vi "Deaktivate HovaCAL MFC Komp fix.vi"(8 "error in (no error)":errorcluster caption="Fehler (Eingang, kein Fehler)", 11 "AutoLin MFC":i32) -> (0 "error out":errorcluster caption="Fehler (Ausgang)", 3 "AutoLin MFC out":i32)   [LabVIEW 2020, in "Linearisierung v2.lvlib" / "Gasteiler.lvlib" / "HovaCAL_Interface.lvlib" / "Helper.lvlib"]
uses:
  Helper.lvlib
  Kommunikation/Kommunikation.lvlib
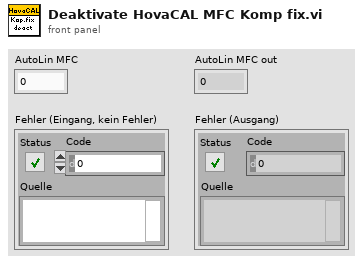
[diagram p1: front panel]
types:
  T1 = cluster{"MFC Komponenten Array":refnum<vi>[], "MFC fix + Array":refnum<vi>[]}
  T2 = enum8{"Enabled", "Disabled", "Disabled and Grayed Out"}
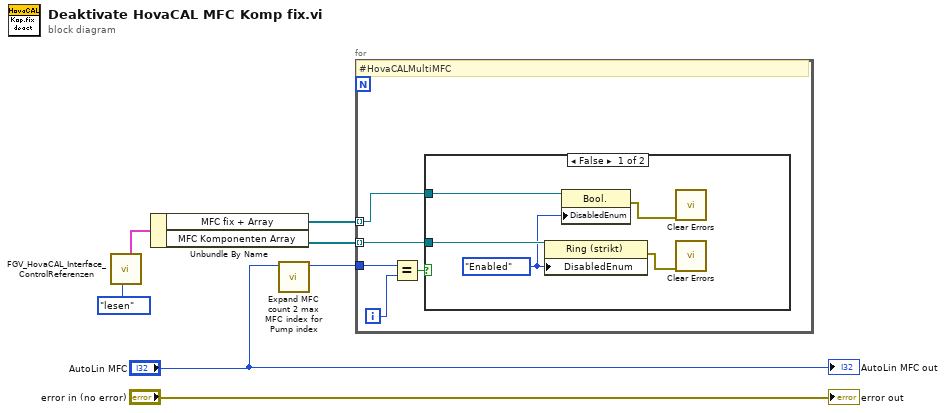
[diagram p0: block diagram]
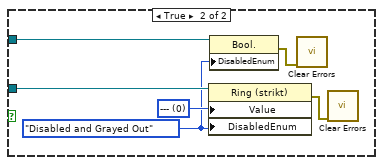
[diagram p2: hidden frame]
diagram:
  n1 = call "FGV_HovaCAL_Interface_ControlReferenzen.vi"("Aktion"=enum16{"lesen", "schreiben"}."lesen") -> ("MFC fix Cluster out"=w5:T1)  [unwired: 6 in, 4 out]
  n2 = Unbundle By Name(w5) -> ("MFC fix + Array"=w3:refnum<vi>[], "MFC Komponenten Array"=w4:refnum<vi>[])
  n3 = call "Expand MFC count 2 max MFC index for Pump index.vi"("AutoLin MFC"="AutoLin MFC") -> ("MFC idx"=w2:i32)  [unwired: 8 in, 2 out]
  n4 = for {
    tunnel: w4 -> [w12] mode=indexing
    tunnel: w2 -> [w11]
    tunnel: w3 -> [w8] mode=indexing
    i -> [w10]
    # "#HovaCALMultiMFC"
    n5 = Equal?(x=w11, y=w10) -> (x = y?=w9:bool)
    n6 = case shown="False" w9 {
      tunnel: w12 -> [w17 w23]
      tunnel: w8 -> [w15 w20]
      frame False {
        w13 = T2."Enabled" ("Deaktiviert")
        n7 = property class="Ring (strikt)"(reference=w17, "DisabledEnum"=w13) -> (error out=w16:errorcluster)  [unwired: 1 in, 1 out]
        n8 = property class="Bool."(reference=w15, "DisabledEnum"=w13) -> (error out=w14:errorcluster)  [unwired: 1 in, 1 out]
        n9 = call <vilib>:"Clear Errors.vi"("error in (no error)"=w14) -> ()  [unwired: 5 in, 2 out]
        n10 = call <vilib>:"Clear Errors.vi"("error in (no error)"=w16) -> ()  [unwired: 5 in, 2 out]
      }
      frame True {
        w18 = T2."Disabled and Grayed Out" ("Deaktiviert")
        w22 = u16 0 items=["---", "NO (350,3000) LP 191C", "NO2 (150) LP 191C (1of2)", "NO2 (2000) LP 191C (2of2)", "N2O (300) LP 191C (1of2)", "NH3 (300) LP 191C (1of2)", "NH3 (900,3000) LP 191C (2of2)", "HNCO (400) 191C", "H2O% (30) LP 191C", "Formaldehyde (70,500) LP 191C", "CO2 low% (4) LP 191C (2of2)", "CO2% (20) LP 191C (1of2)", "CO (700) LP 191C (1of3)", "CO% (1) LP 191C (2of3)", "Propylene (1000) LP 191C", "Aromatic HC C7 (500) LP 191C", "Ethylene (1000) LP 191C", "CH4 (250) LP 191C (1of2)", "CH4 (5000) LP 191C (2of2)", "Ethane (1000) LP 191C", "Acetylene (1000) LP 191C", "HNO2 (20) 191C", "MeOH (1000) 191C", "CO% (10) LP 191C (3of3)", "Formic Acid (100) 191C", "SO2 (500) LP 191C", "Acetaldehyde (1000) LP 191C", "COS (100) LP 191C", "1,3 butadiene (100) LP 191C", "Oil as Octane (200) LP 191C", "N2O (1000) LP 191C (2of2)", "Propane (200) LP 191C", "NO2 autorange (2000)", "CO autorange (100000)", "CH4 autorange (5000)", "NH3 autorange (3000)", "NOx autorange (3000)", "HCD (10000)", "NMHCD (10000)", "CO2% autorange (20)", "H2Oppm (300000)", "N2O autorange (1000)", "NMNEHCD (3000)", "Temp. Gascell", "Pressure Gascell", "sBeam@2500", "Temp. HL zu FT-IR", "Temp. HL Extern SP1", "Austrittstemp. FT-IR", "Temp. Schaltschrank", "Konstant 0", "Konstant 50", "Konstant 100", "AK DUMMY"] ("passive Komponente:")
        n11 = property class="Ring (strikt)"(reference=w23, "Value"=w22, "DisabledEnum"=w18) -> (error out=w21:errorcluster)  [unwired: 1 in, 1 out]
        n12 = property class="Bool."(reference=w20, "DisabledEnum"=w18) -> (error out=w19:errorcluster)  [unwired: 1 in, 1 out]
        n13 = call <vilib>:"Clear Errors.vi"("error in (no error)"=w19) -> ()  [unwired: 5 in, 2 out]
        n14 = call <vilib>:"Clear Errors.vi"("error in (no error)"=w21) -> ()  [unwired: 5 in, 2 out]
      }
    }
  }
  "error out" <- "error in (no error)"
  "AutoLin MFC out" <- "AutoLin MFC"
